vi "MANUAL ARM CONTROLS.vi"(8 "error in (no error)":errorcluster, 9 "Array Joystick axes":dbl[][](array[numeric]), 10 "Array SparkMax DevRef":T1[](array[typedef]), 11 "Array Falcon DevRef":T1[](array[typedef])) -> (0 "error out":errorcluster)   [LabVIEW 2020]
uses:
  <vilib>/Rock Robotics/WPI/MotorControl/WPI_MotorControlDeviceRef.ctl
  <vilib>/Rock Robotics/WPI/MotorControl/WPI_MotorControlType.ctl
  <vilib>/Rock Robotics/SystemInterfaces/DIO/FPGA_DIOPWMChannel.ctl
  <vilib>/Rock Robotics/WPI/PWM/WPI_PWMDeadband.ctl
  <vilib>/Rock Robotics/SystemInterfaces/DIO/FPGA_DIOChannel.ctl
  <vilib>/Rock Robotics/WPI/ThirdParty/Phoenix-LabVIEW/Motor Controller/Controls/CTRE_Phoenix_MotorControl_ControlMode.ctl
  <vilib>/Rock Robotics/WPI/ThirdParty/Phoenix-LabVIEW/Motor Controller/Get/CTRE_Phoenix_MotorController_GetSelectedSensorData.vi
panel:
  out "Velocity (Raw Sensor Units per 100 ms)":i32[](array[numeric])
  out "Position (Raw Sensor Units)":i32[](array[numeric])
  out "Sensor Position":dbl[](array[numeric])
  out "Timestamp":u32[](array[numeric])
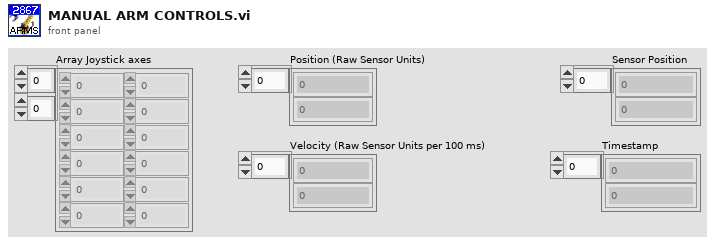
[diagram p1: front panel]
types:
  T1 = typedef "WPI_MotorControlDeviceRef.ctl" = cluster{"DeviceStatus":errorcluster, "Type":T2, "PWM":cluster{"PWM Channel":T3, "DeadBand":T4}, "CAN":cluster{"Device Number":u8, "SetOutput VI Ref":variant, "GetOutput VI Ref":variant, "Enable VI Ref":variant, "Disable VI Ref":variant, "Data":variant}, "Invert":bool, "DIO PWM":cluster{"PWM \"Enable\" Channel":T3, "DIOChannel":T5, "PWM Rate":dbl}}
  T2 = typedef "WPI_MotorControlType.ctl" = enum16{"PWM", "CAN", "DIO PWM"}
  T3 = typedef "FPGA_DIOPWMChannel.ctl" = enum8{"PWM 0", "PWM 1", "PWM 2", "PWM 3", "PWM 4", "PWM 5", "PWM 6", "PWM 7", "PWM 8", "PWM 9", "PWM MXP 0", "PWM MXP 1", "PWM MXP 2", "PWM MXP 3", "PWM MXP 4", "PWM MXP 5", "PWM MXP 6", "PWM MXP 7", "PWM MXP 8", "PWM MXP 9", "Invalid"}
  T4 = typedef "WPI_PWMDeadband.ctl" = cluster{"Name":string, "maxPositivePwm":i32, "minPositivePwm":i32, "centerPwm":i32, "maxNegativePwm":i32, "minNegativePwm":i32, "angularRange":u16}
  T5 = typedef "FPGA_DIOChannel.ctl" = enum8{"DIO 0", "DIO 1", "DIO 2", "DIO 3", "DIO 4", "DIO 5", "DIO 6", "DIO 7", "DIO 8", "DIO 9", "DIO MXP 0", "DIO MXP 1", "DIO MXP 2", "DIO MXP 3", "DIO MXP 4", "DIO MXP 5", "DIO MXP 6", "DIO MXP 7", "DIO MXP 8", "DIO MXP 9", "DIO MXP 10", "DIO MXP 11", "DIO MXP 12", "DIO MXP 13", "DIO MXP 14", "DIO MXP 15", "SPI Port CS1", "SPI Port CS2", "SPI Port CS3", "SPI Port MISO", "SPI Port MOSI", "Invalid"}
  T6 = typedef "CTRE_Phoenix_MotorControl_ControlMode.ctl" = u16
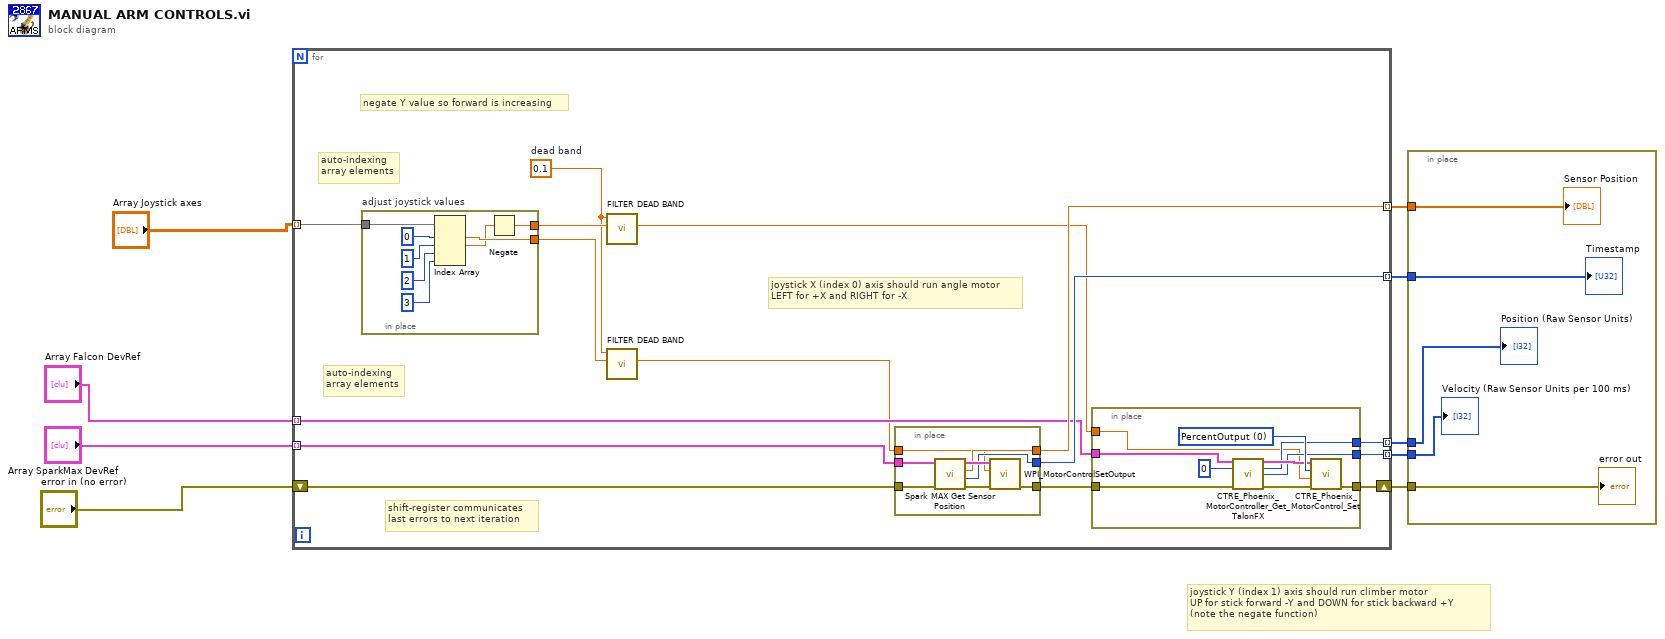
[diagram p0: block diagram]
diagram:
  # "joystick Y (index 1) axis should run climber motor\nUP for stick forward -Y and DOWN for stick backward +Y\n(note the negate function)"
  n1 = for {
    tunnel: "Array Joystick axes" -> [w24] mode=indexing
    shift-right: [w21] -> w8
    shift-left: "error in (no error)" -> [w20]
    tunnel: [w18] -> w7 mode=indexing
    tunnel: [w17] -> w6 mode=indexing
    tunnel: [w16] -> w5 mode=indexing
    tunnel: [w15] -> w4 mode=indexing
    tunnel: "Array Falcon DevRef" -> [w13] mode=indexing
    tunnel: "Array SparkMax DevRef" -> [w12] mode=indexing
    w14 = 0.1  # dead band
    # "negate Y value so forward is increasing"
    # "auto-indexing\narray elements"
    # "auto-indexing\narray elements"
    # "joystick X (index 0) axis should run angle motor\nLEFT for +X and RIGHT for -X"
    # "shift-register communicates\nlast errors to next iteration"
    n2 = in-place "adjust joystick values" {
      in-place-border: w24 -> [w50]
      in-place-border: [w45] -> w23
      in-place-border: [w43] -> w22
      n3 = Index Array(array=w50, index #1=0 ("index"), index #2=1 ("index"), index #3=2 ("index"), index #4=3 ("index")) -> (element #1=w45:dbl, element #2=w44:dbl)  [unwired: 2 out]
      n4 = Negate(x=w44) -> (-x=w43:dbl)
    }
    n5 = call "FILTER DEAD BAND.vi"("Joystick value in"=w22, "dead band%"=w14) -> ("Joystick value out"=w10:dbl)  [unwired: 8 in, 1 out]
    n6 = call "FILTER DEAD BAND.vi"("Joystick value in"=w23, "dead band%"=w14) -> ("Joystick value out"=w11:dbl)  [unwired: 8 in, 1 out]
    n7 = in-place {
      in-place-border: w12 -> [w32]
      in-place-border: w20 -> [w30]
      in-place-border: [w28] -> w19
      in-place-border: [w27] -> w16
      in-place-border: [w26] -> w15
      in-place-border: w11 -> [w25]
      n8 = call <vilib>:"Spark MAX Get Sensor Position.vi"("error in (no error)"=w30, "MotorControlDevRef in"=w32) -> ("error out"=w29:errorcluster, "Timestamp"=w27:u32, "Sensor Position"=w26:dbl, "MotorControlDevRef out"=w31:T1)  [unwired: 6 in]
      n9 = call <vilib>:"WPI_MotorControlSetOutput.vi"("error in (no error)"=w29, "Output"=w25, "MotorControlDevRef"=w31) -> ("error out"=w28:errorcluster)  [unwired: 6 in, 2 out]
    }
    n10 = in-place {
      in-place-border: w13 -> [w42]
      in-place-border: [w40] -> w21
      in-place-border: w19 -> [w36]
      in-place-border: [w35] -> w18
      in-place-border: [w34] -> w17
      in-place-border: w10 -> [w33]
      w41 = T6 0 items=["PercentOutput"=0, "Position"=1, "Velocity"=2, "Current"=3, "Follower"=5, "MotionProfile"=6, "MotionMagic"=7, "MotionProfileArc"=10, "Disabled"=15] ("Control Mode")
      n11 = call-poly <vilib>:"CTRE_Phoenix_MotorController_Get_TalonFX.vi"("PhoenixMotorControlDevRef"=w42, "pidLoopIdx"=u32 0, "error in"=w36) -> ("PhoenixMotorControlDevRef"=w39:T1, "Position (Raw Sensor Units)"=w35:i32, "Velocity (Raw Sensor Units per 100 ms)"=w34:i32, "error out"=w37:errorcluster)  [unwired: 9 in]
      n12 = call <vilib>:"CTRE_Phoenix_MotorControl_Set.vi"("error in (no error)"=w37, "Output"=w33, "Control Mode"=w41, "PhoenixMotorControlDevRef"=w39) -> ("error out"=w40:errorcluster)  [unwired: 6 in, 1 out]
    }
  }
  n13 = in-place {
    in-place-border: w8 -> [w55]
    in-place-border: w7 -> [w54]
    in-place-border: w6 -> [w53]
    in-place-border: w5 -> [w52]
    in-place-border: w4 -> [w51]
    "error out" <- w55
    "Position (Raw Sensor Units)" <- w54
    "Velocity (Raw Sensor Units per 100 ms)" <- w53
    "Timestamp" <- w52
    "Sensor Position" <- w51
  }
